vi "ProcessName.vi"() -> (1 "process name":string)   [LabVIEW 2017, in "CmsTestPanel.lvlib"]
uses:
  <vilib>/addons/InsightCM/Devices/Shared/Cms/CmsTestPanel/CmsTestPanel.lvlib
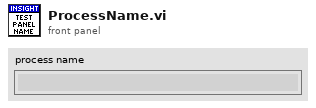
[diagram p1: front panel]
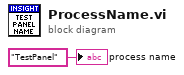
[diagram p0: block diagram]
diagram:
  "process name" <- "TestPanel" ("ProcessName")
